vi "Convert to Postive 360 Angle.vi"(11 "Angle in":dbl) -> (3 "Angle out":dbl)   [LabVIEW 2016]
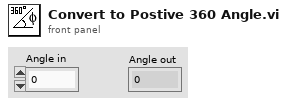
[diagram p1: front panel]
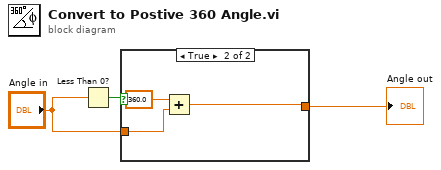
[diagram p0: block diagram]
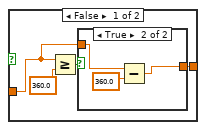
[diagram p2: hidden frame]
diagram:
  n1 = Less Than 0?(x="Angle in") -> (x < 0?=w1:bool)
  n2 = case shown="True" w1 {
    tunnel: "Angle in" -> [w5 w14]
    tunnel: [w4 w12] -> w3
    frame False {
      n3 = Greater Or Equal?(x=w5, y=360.0) -> (x >= y?=w6:bool)
      n4 = case shown="True" w6 {
        tunnel: w5 -> [w8 w10]
        tunnel: [w8 w9] -> w4
        frame False {
        }
        frame True {
          n5 = Subtract(x=w10, y=360.0) -> (x-y=w9:dbl)
        }
      }
    }
    frame True {
      n6 = Add(x=360.0, y=w14) -> (x+y=w12:dbl)
    }
  }
  "Angle out" <- w3
